vi "Set Report Margins.vi"(4 "error in (no error)":errorcluster, 5 "measurement system (Default)":u16(ring) items=["Default", "US", "Metric"], 6 "margins (1.00)":T2={"top"=1.0, "left"=1.0, "right"=1.0, "bottom"=1.0} {"right" format="%.2f"; "bottom" format="%.2f"; "top" format="%.2f"; "left" format="%.2f"}, 7 "report in":T1) -> (0 "error out":errorcluster, 3 "report out":T1)   [LabVIEW 2015]
doc: "Sets the margins of the specified report."
uses:
  <vilib>/Utility/NIReport.llb/Generate Report Object Reference.ctl
  <vilib>/Utility/NIReport.llb/NI_report.lvclass
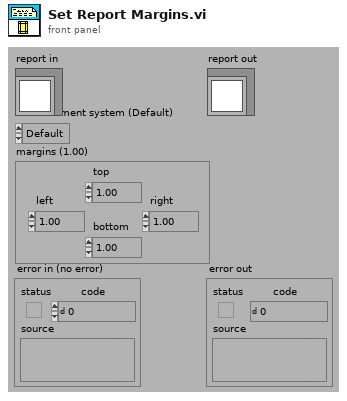
[diagram p1: front panel]
types:
  T1 = typedef "Generate Report Object Reference.ctl" = refnum<class "NI_report.lvclass">
  T2 = cluster{"top":dbl, "left":dbl, "right":dbl, "bottom":dbl}
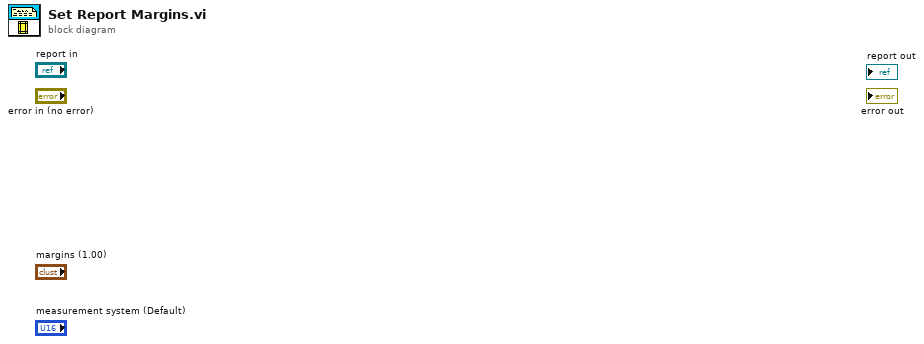
[diagram p0: block diagram]
diagram:
